vi "WriteAttributeTest.vi"() -> ()   [LabVIEW 2013, in "examples.lvlib"]
uses:
  examples.lvlib
  vis/lv-2013/tango_vi.llb/_TangoWriteStringScalarAttribute.vi
  vis/lv-2013/tango_vi.llb/_TangoWriteShortScalarAttribute.vi
  vis/lv-2013/tango_vi.llb/_TangoWriteLongScalarAttribute.vi
  vis/lv-2013/tango_vi.llb/_TangoWriteDoubleScalarAttribute.vi
  vis/lv-2013/tango_vi.llb/tango.lvlib
panel:
  out "success":bool
  out "success":bool
  out "success":bool
  out "success":bool
  in  "value":dbl=123.456
  in  "attribute name":string="double_scalar"
  in  "value":i32=1550
  in  "attribute name":string="long_scalar"
  in  "value":i16=256
  in  "attribute name":string="short_scalar"
  in  "value":string="This is the write value..."
  in  "attribute name":string="string_scalar"
  in  "device name":string="sys/tg_test/1"
  # "TANGO  Binding for LabVIEW - Write Attribute Example"
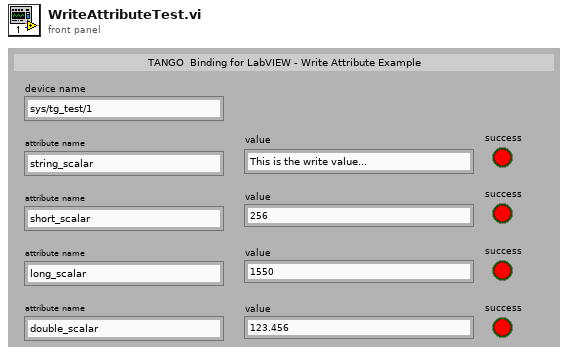
[diagram p1: front panel]
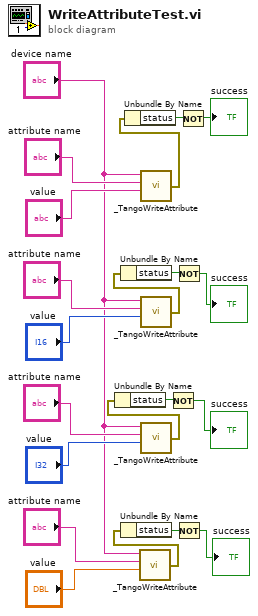
[diagram p0: block diagram]
diagram:
  n1 = call-poly "_TangoWriteAttribute.vi"("value"="value", "attribute name"="attribute name", "device name"="device name") -> ("error out"=w9:errorcluster)  [unwired: 1 in]
  n2 = Unbundle By Name(w9) -> ("status"=w1:bool)
  n3 = call-poly "_TangoWriteAttribute.vi"("value"="value", "attribute name"="attribute name", "device name"="device name") -> ("error out"=w12:errorcluster)  [unwired: 1 in]
  n4 = Unbundle By Name(w12) -> ("status"=w11:bool)
  n5 = call-poly "_TangoWriteAttribute.vi"("value"="value", "attribute name"="attribute name", "device name"="device name") -> ("error out"=w5:errorcluster)  [unwired: 1 in]
  n6 = Unbundle By Name(w5) -> ("status"=w3:bool)
  n7 = call-poly "_TangoWriteAttribute.vi"("value"="value", "attribute name"="attribute name", "device name"="device name") -> ("error out"=w7:errorcluster)  [unwired: 1 in]
  n8 = Unbundle By Name(w7) -> ("status"=w2:bool)
  n9 = Not(x=w2) -> (.not. x?=→"success":bool)
  n10 = Not(x=w3) -> (.not. x?=→"success":bool)
  n11 = Not(x=w1) -> (.not. x?=→"success":bool)
  n12 = Not(x=w11) -> (.not. x?=→"success":bool)
